vi "Get Current State.vi"(7 "Additional Reply Message Queues (Default 0)":i32, 8 "error in (no error)":errorcluster, 11 "API-Reference in":refnum<data-value>) -> (0 "error out":errorcluster, 1 "Additional Reply Message References":refnum<event-registration>[](array[refnum]), 2 "Current State":refnum<event-registration>, 3 "API-Reference out":refnum<data-value>)   [LabVIEW 2018, in "Scripting.lvlib" / "Actor.lvclass"]
uses:
  Actor.lvclass
  API-Data.ctl
  Front-Panel State.ctl
  Did Stop.ctl
  All-Enqueuers.ctl
  Broadcast Enqueuers.ctl
  Did Initialize.ctl
  Request-Enqueuers.ctl
  Get State.ctl
  State.ctl
  Stop.ctl
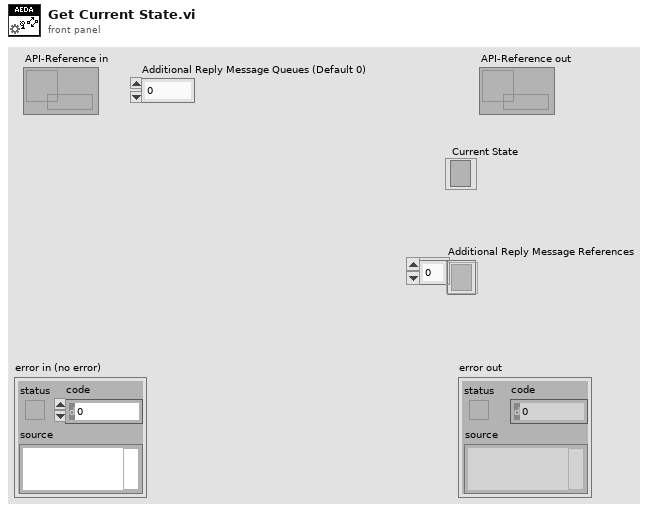
[diagram p1: front panel]
types:
  T1 = typedef "Scripting.lvlib/Actor.lvclass/Get State.ctl" = cluster{"Reply":refnum<user-event>}
  T2 = typedef "Scripting.lvlib/Actor.lvclass/API-Data.ctl" = cluster{"Launch":refnum<notifier>, "Did Stop Message":refnum<event-registration>, "Did Stop Enqueuer":refnum<user-event>, "Enqueuers":T3}
  T3 = typedef "Scripting.lvlib/Actor.lvclass/All-Enqueuers.ctl" = cluster{"Broadcasts":T4, "Requests":T5}
  T4 = typedef "Scripting.lvlib/Actor.lvclass/Broadcast Enqueuers.ctl" = cluster{"Did Initialize":refnum<user-event>}
  T5 = typedef "Scripting.lvlib/Actor.lvclass/Request-Enqueuers.ctl" = cluster{"Get State":refnum<user-event>, "Stop":refnum<user-event>}
  T6 = typedef "Scripting.lvlib/Actor.lvclass/State.ctl" = cluster{"Current State":refnum<class "Actor.lvclass">}
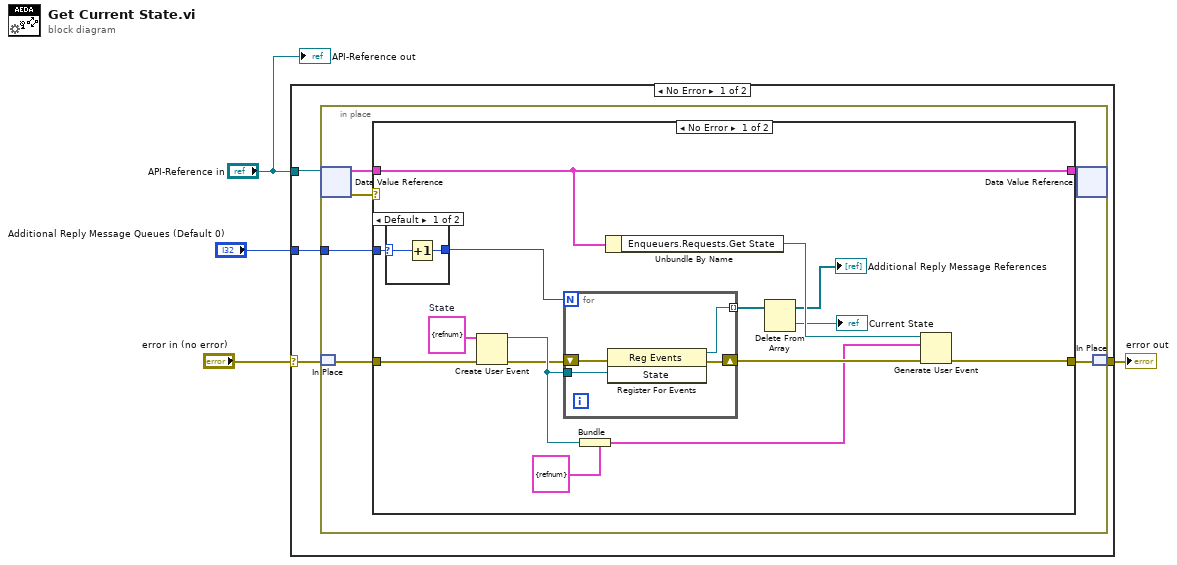
[diagram p0: block diagram]
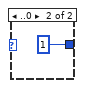
[diagram p2: hidden frame]
diagram:
  n1 = case shown="No Error" "error in (no error)" {
    selector: "error in (no error)" -> [w8 w39]
    tunnel: [w7 w39] -> w3
    tunnel: "API-Reference in" -> [w6 _]
    tunnel: "Additional Reply Message Queues (Default 0)" -> [w5 _]
    frame No Error {
      n2 = in-place {
        in-place-border: w5 -> [w9]
        n3 = in-place-dvr #1(w6) -> (w13:T2, w14:errorcluster)
        n4 = in-place-match #2(w8) -> (w11:errorcluster)
        n5 = case shown="No Error" w14 {
          selector: w14 -> [_ w38]
          tunnel: w13 -> [w29 w37]
          tunnel: [w29 w37] -> w12
          tunnel: w11 -> [w28 _]
          tunnel: [w26 w38] -> w10
          tunnel: w9 -> [w23 _]
          frame No Error {
            w19 = T6 {"Current State"=refnum}  # State
            n6 = case shown="Default" w23 {
              selector: w23 -> [w31 _]
              tunnel: [w30 1] -> w22
              frame Default {
                n7 = Increment(x=w31) -> (x+1=w30:i32)
              }
              frame ..0 {
              }
            }
            n8 = Create User Event(user event datatype=w19, error in=w28) -> (user event=w24:refnum<user-event>, error out=w21:errorcluster)
            n9 = for {
              N: w22 -> [_]
              shift-right: [w35] -> w27
              shift-left: w21 -> [w36]
              tunnel: [w34] -> w20 mode=indexing
              tunnel: w24 -> [w33]
              n10 = register-events(error in=w36, w33) -> (reference out=w34:refnum<event-registration>, error out=w35:errorcluster)  [unwired: 1 in]
            }
            n11 = Bundle(cluster=T1 {"Reply"=refnum} ("Get State"), "Reply"=w24) -> (w17:T1)
            n12 = Unbundle By Name(w29) -> ("Enqueuers.Requests.Get State"=w25:refnum<user-event>)
            n13 = Delete From Array(array=w20) -> (deleted portion=→"Current State":refnum<event-registration>, array with subset deleted=→"Additional Reply Message References":refnum<event-registration>[])  [unwired: 2 in]
            n14 = Generate User Event(user event=w25, event data cluster=w17, error in=w27) -> (error out=w26:errorcluster)  [unwired: 1 in, 1 out]
          }
          frame Error {
          }
        }
        n15 = in-place-dvr #1(w12) -> ()  [unwired: 2 out]
        n16 = in-place-match #2(w10) -> (w7:errorcluster)
      }
    }
    frame Error {
    }
  }
  "error out" <- w3
  "API-Reference out" <- "API-Reference in"
